vi "Calibration_VI.vi"() -> ()   [LabVIEW 2020]
uses:
  <vilib>/Analysis/baseanly.llb/Mean (DBL).vi
  <vilib>/Analysis/NI_AALBase.lvlib
panel:
  in  "Time to run the Motor":dbl=1.0 format="%#_13g"
  in  "Start Recording Data":bool
  in  "Pressure displayed in Omron [mmHg]":dbl
  in  "Omron Ready ?":bool
  in  "Stop Expt":bool caption="Stop Experiment"
  out "Mean DC Voltage":dbl format="%0.2f"
  in  "Stop Recording Data":bool
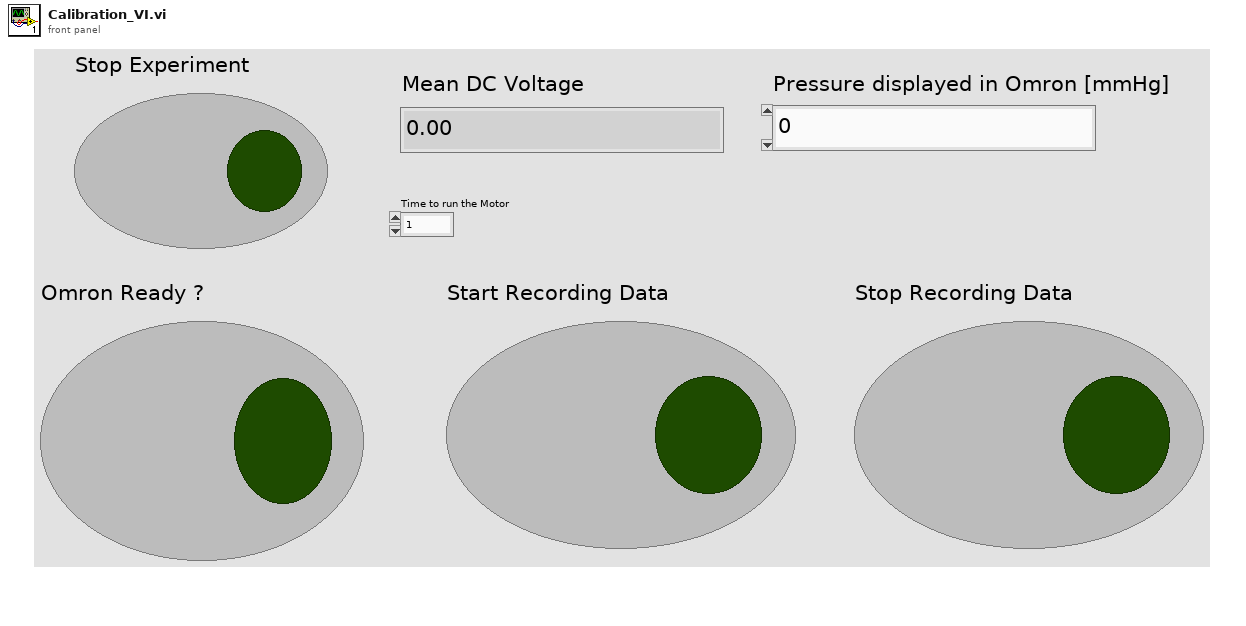
[diagram p1: front panel]
types:
  T1 = enum16{"Increase Pressure", "Reduce Pressure", "Hold Pressure", "Zero State (Omron)"}
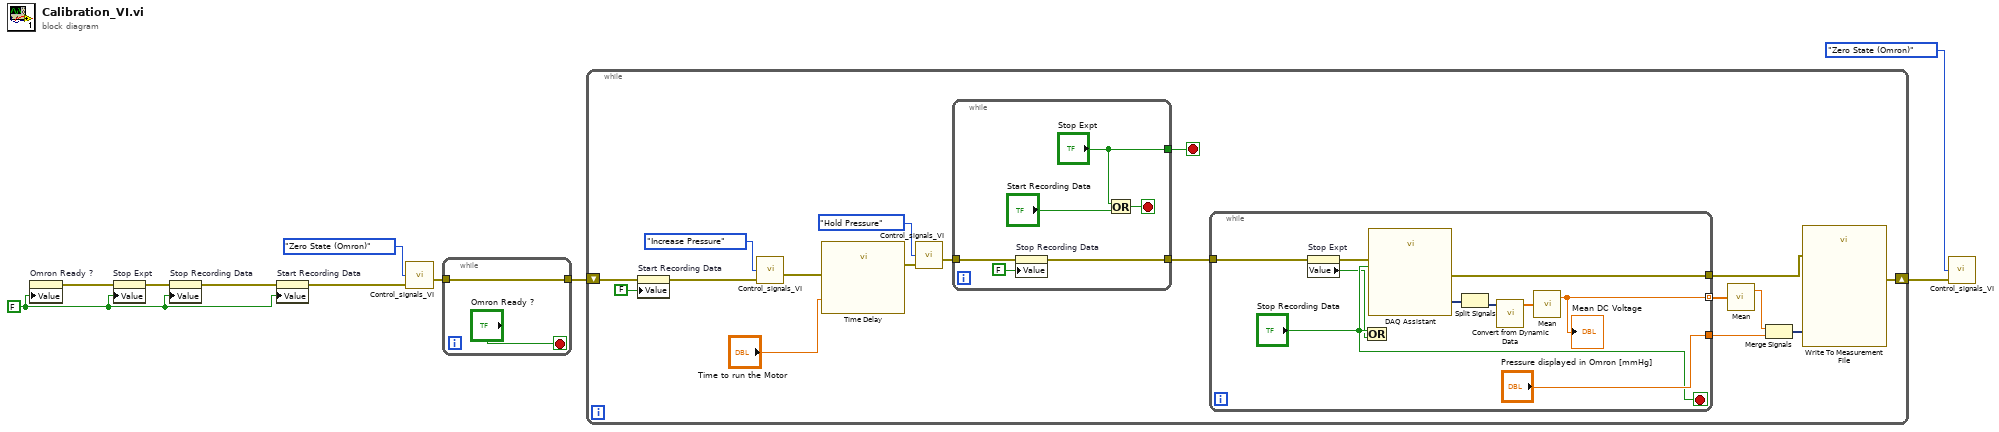
[diagram p0: block diagram]
diagram:
  w4 = FALSE
  n1 = property on="Omron Ready ?" class="Bool (strict)"("Value"=w4) -> (error out=w5:errorcluster)  [unwired: 2 in, 1 out]
  n2 = property on="Stop Expt" class="Bool (strict)"(error in=w5, "Value"=w4) -> (error out=w3:errorcluster)  [unwired: 1 in, 1 out]
  n3 = property on="Stop Recording Data" class="Bool (strict)"(error in=w3, "Value"=w4) -> (error out=w2:errorcluster)  [unwired: 1 in, 1 out]
  n4 = property on="Start Recording Data" class="Bool (strict)"(error in=w2, "Value"=w4) -> (error out=w1:errorcluster)  [unwired: 1 in, 1 out]
  n5 = call "Control_signals_VI.vi"("Input"=T1."Zero State (Omron)", "error in"=w1) -> ("error out"=w8:errorcluster)  [unwired: 4 in, 1 out]
  n6 = while {
    tunnel: w8 -> [w12]
    tunnel: [w12] -> w7
    stop <- "Omron Ready ?" stop-if-true
  }
  n7 = while {
    shift-right: [w23] -> w9
    shift-left: w7 -> [w19]
    stop <- w13 stop-if-true
    n8 = property on="Start Recording Data" class="Bool (strict)"(error in=w19, "Value"=FALSE) -> (error out=w18:errorcluster)  [unwired: 1 in, 1 out]
    n9 = call "Control_signals_VI.vi"("Input"=T1."Increase Pressure", "error in"=w18) -> ("error out"=w27:errorcluster)  [unwired: 4 in, 1 out]
    n10 = call "Time Delay"("error in (no error)"=w27, "Delay Time (s)"="Time to run the Motor") -> ("error out"=w16:errorcluster)  [unwired: 9 in]
    n11 = call "Control_signals_VI.vi"("Input"=T1."Hold Pressure", "error in"=w16) -> ("error out"=w15:errorcluster)  [unwired: 4 in, 1 out]
    n12 = while {
      tunnel: w15 -> [w35]
      tunnel: [w34] -> w14
      tunnel: ["Stop Expt"] -> w13
      stop <- w30 stop-if-true
      n13 = property on="Stop Recording Data" class="Bool (strict)"(error in=w35, "Value"=FALSE) -> (error out=w34:errorcluster)  [unwired: 1 in, 1 out]
      n14 = Or(x="Stop Expt", y="Start Recording Data") -> (x .or. y?=w30:bool)
    }
    n15 = while {
      tunnel: [w44] -> w24
      tunnel: [w41] -> w28 mode=indexing
      tunnel: ["Pressure displayed in Omron [mmHg]"] -> w20
      tunnel: w14 -> [w37]
      stop <- "Stop Recording Data" stop-if-true
      n16 = property on="Stop Expt" class="Bool (strict)"(error in=w37) -> (error out=w36:errorcluster, "Value"=w38:bool)  [unwired: 1 in, 1 out]
      n17 = Or(x="Stop Recording Data", y=w38) -> ()  [unwired: 1 out]
      n18 = call "DAQ Assistant"("error in"=w36, "stop (T)"="Stop Recording Data") -> ("data"=w45:dynamicdata, "error out"=w44:errorcluster)  [unwired: 15 in, 1 out]
      n19 = Split Signals(w45) -> (w43:dynamicdata)  [unwired: 2 in, 1 out]
      n20 = call "Convert from Dynamic Data"("Dynamic Data Type"=w43) -> ("Array"=w42:dbl[])  [unwired: 3 in]
      n21 = call-poly <vilib>:"Mean.vi"("X"=w42) -> ("mean"=w41:dbl)  [unwired: 1 out]
      "Mean DC Voltage" <- w41
    }
    n22 = call-poly <vilib>:"Mean.vi"("X"=w28) -> ("mean"=w22:dbl)  [unwired: 1 out]
    n23 = Merge Signals(w22, w20) -> (w21:dynamicdata)
    n24 = call "Write To Measurement File"("Signals"=w21, "error in (no error)"=w24) -> ("error out"=w23:errorcluster)  [unwired: 15 in, 2 out]
  }
  n25 = call "Control_signals_VI.vi"("Input"=T1."Zero State (Omron)", "error in"=w9) -> ()  [unwired: 4 in, 2 out]
